vi "rest_get_history.vi"(8 "error in (no error)":errorcluster, 11 "Base URL":string="http://localhost:5001/") -> (0 "error out":errorcluster, 7 "String":T1)   [LabVIEW 2024]
uses:
  TypeDefs/Control 1.ctl
  <vilib>/addons/_JKI.lib/REST Client/classes/REST Client/REST Client.lvclass
panel:
  out "Response body":string
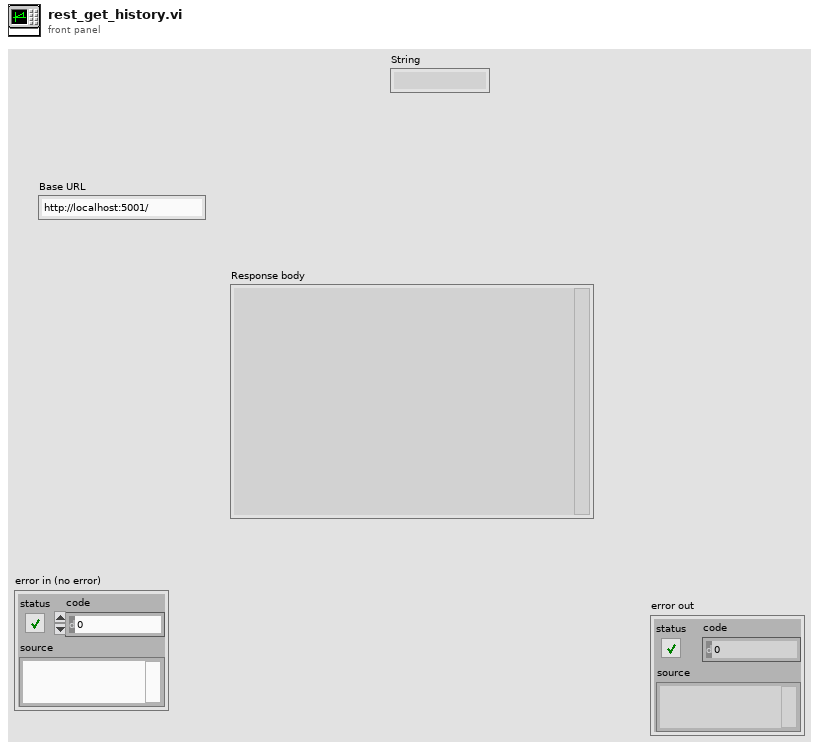
[diagram p1: front panel]
types:
  T1 = typedef "Control 1.ctl" = string
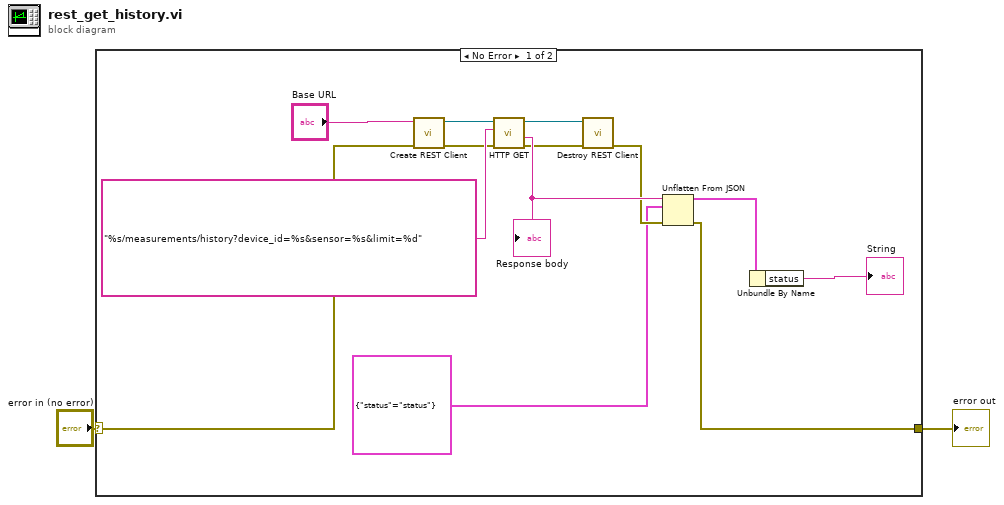
[diagram p0: block diagram]
diagram:
  n1 = case shown="No Error" "error in (no error)" {
    selector: "error in (no error)" -> [w10 w16]
    tunnel: [w6 w16] -> w1
    frame No Error {
      n2 = call <vilib>:"Create REST Client.vi"("error in (no error)"=w10, "Base URL"="Base URL") -> ("error out"=w9:errorcluster, "REST Client out"=w15:refnum<class "REST Client.lvclass">)  [unwired: 8 in]
      n3 = call-dynamic "HTTP GET.vi"("error in (no error)"=w9, "Path"="%s/measurements/history?device_id=%s&sensor=%s&limit=%d", "REST Client in"=w15) -> ("error out"=w8:errorcluster, "Response body"=w11:string, "REST Client out"=w14:refnum<class "REST Client.lvclass">)  [unwired: 3 in, 3 out]
      "Response body" <- w11
      n4 = call-dynamic "Destroy REST Client.vi"("error in (no error)"=w8, "REST Client in"=w14) -> ("error out"=w7:errorcluster)  [unwired: 9 in]
      n5 = Unflatten From JSON(JSON string=w11, type and defaults=cluster{"status":T1} {"status"="status"}, error in (no error)=w7) -> (value=w4:cluster{"status":T1}, error out=w6:errorcluster)  [unwired: 4 in]
      n6 = Unbundle By Name(w4) -> ("status"=→"String":T1)
    }
    frame Error {
    }
  }
  "error out" <- w1
